vi "CPP_TubingCorrectionFromCrossSpectra.vi"() -> (5 "Plug in titles":string[](array[string]), 7 "Plug in values":string[](array[string]))   [LabVIEW 2010]
uses:
  Globals/Meas_global.vi
  Globals/Plug_in_data_global.vi
  <vilib>/Analysis/NI_AALPro.lvlib
  <vilib>/Analysis/NI_AALBase.lvlib
panel:
  out "CutoffFrequencyUsed":dbl=15.0
  out "MaxBoostUsed":dbl=15.0
  in  "CutoffFrequency":dbl=200.0
  in  "MaxBoost":dbl=15.0
  out "TimeSeries":T1(graph)
  in  "Ref":u16(ring) items=["RV (Amp)"]
  in  "Test":u16(ring) items=["RV (Amp)"]
  out "Spectra":cluster{dbl, dbl, dbl[][]}(graph)
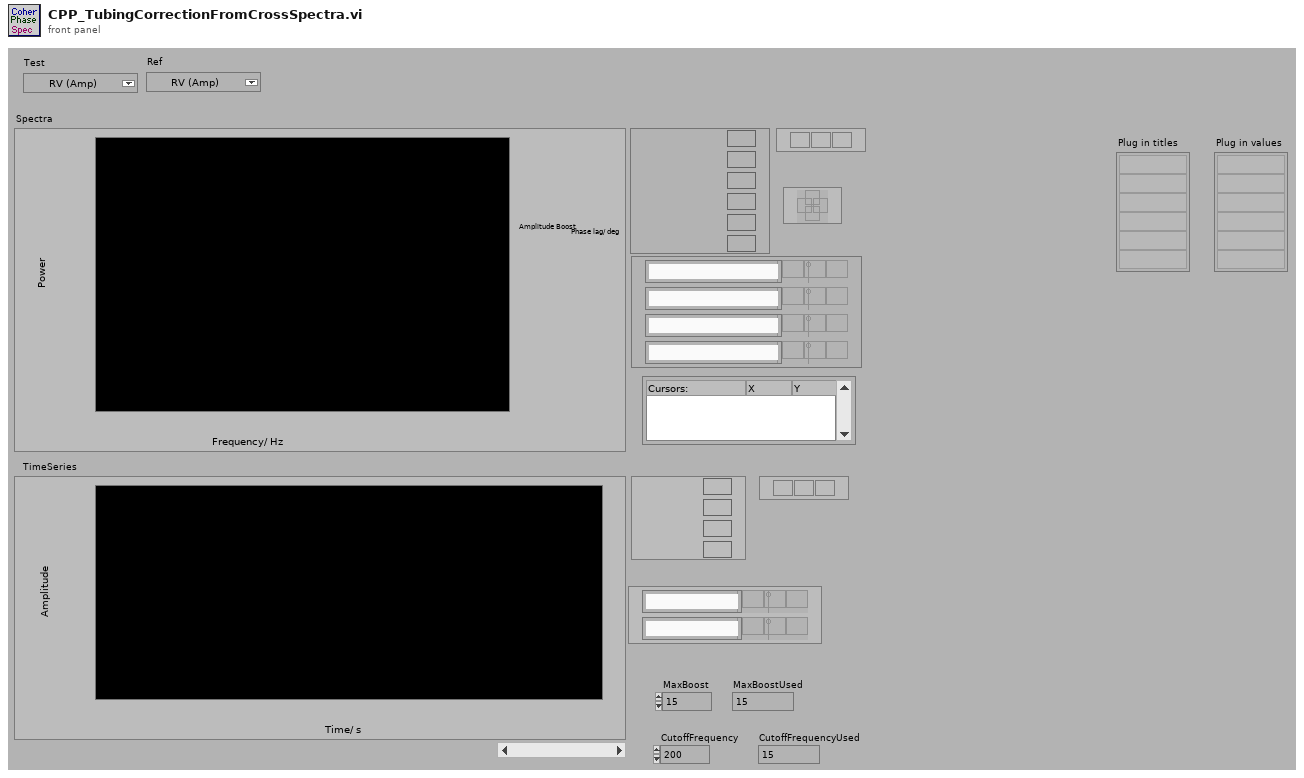
[diagram p1: front panel]
types:
  T1 = cluster{dbl, "Actual Sampling rate (Hz)":dbl, dbl[][]}
  T2 = typedef "Analysis_info_cluster.ctl" = cluster{"Colour":u32, "Inst type":T3, "Inst name":string, "Symbol":string, "Code name":string, "Extra Info":string, "Inst Array":T4, "Index":i32, "Voltage Index":i32, "Extra Titles":string[], "Extra Values":string[]}
  T3 = typedef "Inst_type.ctl" = enum16{"Propeller anemometer", "Raw voltage", "Pressure Transducer", "Pitot-static tube", "Preston tube", "Hot wire", "Cross wire 1", "Cross wire 2", "Generic Linear", "Generic Polynomial", "Generic BackPoly", "Fast FID", "Thermocouple", "Cold wire", "Pulsed Wire", "LDA Vel", "LDA Tran time", "LDA Arr time"}
  T4 = typedef "Instrument_Array.ctl" = enum16{"PWA", "LDA", "Analogue"}
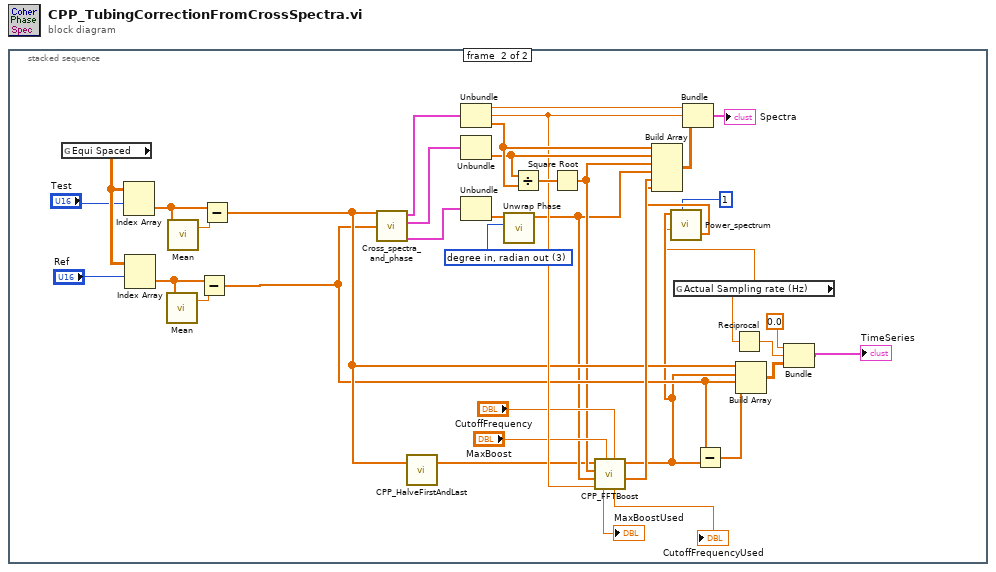
[diagram p0: block diagram]
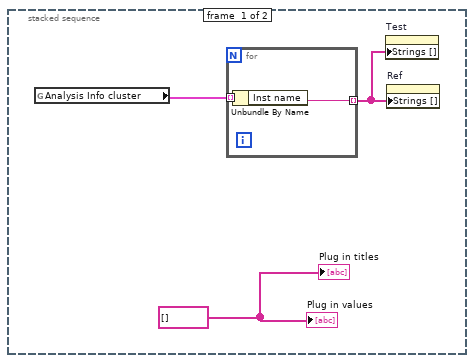
[diagram p2: hidden frame]
diagram:
  n1 = stacked-sequence {
    frame #0 {
      w1 = string[] [] ("Add in values")
      n2 = global read "Meas_global.vi" "Analysis Info cluster"() -> (w3:T2[])
      n3 = for {
        tunnel: w3 -> [w5] mode=indexing
        tunnel: [w4] -> w2 mode=indexing
        n4 = Unbundle By Name(w5) -> ("Inst name"=w4:string)
      }
      n5 = property on="Test" class="Ring (strict)"("Strings []"=w2) -> ()  [unwired: 2 in, 2 out]
      n6 = property on="Ref" class="Ring (strict)"("Strings []"=w2) -> ()  [unwired: 2 in, 2 out]
      "Plug in titles" <- w1
      "Plug in values" <- w1
    }
    frame #1 {
      w31 = 3 items=["radian in, radian out", "radian in, degree out", "degree in, degree out", "degree in, radian out"] ("phase unit")
      n7 = global read "Plug_in_data_global.vi" "Equi Spaced"() -> (w43:dbl[][])
      n8 = Index Array(array=w43, index (row)="Test") -> (element=w22:dbl[])  [unwired: 1 in]
      n9 = Index Array(array=w43, index (row)="Ref") -> (element=w23:dbl[])  [unwired: 1 in]
      n10 = call <vilib>:"Mean.vi"("X"=w23) -> ("mean"=w24:dbl)  [unwired: 1 out]
      n11 = call <vilib>:"Mean.vi"("X"=w22) -> ("mean"=w25:dbl)  [unwired: 1 out]
      n12 = Subtract(x=w23, y=w24) -> (x-y=w13:dbl[])
      n13 = Subtract(x=w22, y=w25) -> (x-y=w14:dbl[])
      n14 = call "Cross_spectra_and_phase.vi"("U1"=w14, "U2"=w13) -> ("U1 spectra"=w40:cluster{dbl, dbl, dbl[]}, "U2 spectra"=w39:cluster{dbl, dbl, dbl[]}, "U1 U2 phase"=w33:cluster{dbl, dbl, "Phase array":dbl[]})  [unwired: 4 out]
      n15 = call "CPP_HalveFirstAndLast.vi"("InputArray"=w14) -> ("HalvedEnds"=w10:dbl[])  [unwired: 2 in]
      n16 = Unbundle(w40) -> (w37:dbl, w20:dbl, w35:dbl[])
      n17 = Unbundle(w39) -> (w34:dbl[])  [unwired: 2 out]
      n18 = Unbundle(w33) -> ("Phase array"=w32:dbl[])  [unwired: 2 out]
      n19 = call <vilib>:"Unwrap Phase.vi"("phase unit"=w31, "Phase"=w32) -> ("Unwrapped Phase"=w11:dbl[])  [unwired: 8 in, 1 out]
      n20 = Divide(x=w34, y=w35) -> (x/y=w26:dbl[])
      n21 = Square Root(x=w26) -> (sqrt(x)=w12:dbl[])
      n22 = call "CPP_FFTBoost.vi"("CutoffFrequency"="CutoffFrequency", "MaxBoost"="MaxBoost", "dF"=w20, "UnwrappedPhaseLag"=w11, "AmplitudeBoost"=w12, "Muffleddata"=w10) -> ("BandLimitedBoost"=w15:dbl[], "boostedData"=w9:dbl[], "CutoffFrequencyUsed"=→"CutoffFrequencyUsed":dbl, "MaxBoostUsed"=→"MaxBoostUsed":dbl)  [unwired: 2 in]
      n23 = global read "Meas_global.vi" "Actual Sampling rate (Hz)"() -> (w7:dbl)
      n24 = call "Power_spectrum.vi"("U"=w9, "Sampling frequency"=w7, "Block No"=1) -> ("Spectrum output array"=w8:dbl[])  [unwired: 2 in, 1 out]
      n25 = Build Array(w35, w34, w12, w11, w15, w8) -> (w38:dbl[][])
      n26 = Bundle(w37, w20, w38) -> (→"Spectra":cluster{dbl, dbl, dbl[][]})  [unwired: 1 in]
      n27 = Subtract(x=w13, y=w9) -> (x-y=w21:dbl[])
      n28 = Reciprocal(x=w7) -> (1/x=w27:dbl)
      n29 = Build Array(w14, w9, w13, w21) -> (w30:dbl[][])
      n30 = Bundle(0.0, w27, w30) -> (→"TimeSeries":cluster{dbl, dbl, dbl[][]})  [unwired: 1 in]
    }
  }
